vi "EncodersTickCount.vi"() -> (0 "Right ccw  total pulse count":i32, 1 "Left ccw  total pulse count":i32, 2 "Right Motor Pulses per 16 mSec":i32, 3 "Left Motor Pulses per 16 mSec":i32)   [LabVIEW 2013]
doc: "This VI implements the low level control of the motors and sensor for the Starter Kit 2.0 robot. The functionality of this VI is similar to the fixed FPGA personality used by the Starter Kit API."
uses:
  <vilib>/Platform/TimedLoop/XDataNode/timing_clust.ctl
  <vilib>/Platform/TimedLoop/XDataNode/nitl_modes.ctl
  <vilib>/Platform/TimedLoop/XDataNode/wakeup.ctl
  <vilib>/robotics/Utilities/Encoder Count Encoding.ctl
  <vilib>/rvi/Emulation/niFpgaSctlEmulationGetInTimedLoop.vi
  <vilib>/rvi/Emulation/niFpgaEmulationReportErrorSimple.vi
  <vilib>/rvi/Emulation/niFpgaGetClockAttributes.vi
  <vilib>/rvi/Emulation/niFpgaCriticalErrorInLSC.vi
  <vilib>/robotics/Utilities/FPGA Utilities/Count Two Phase Digital Encoder.vi
  Support VIs/Starter Kit 2.0 FPGA Globals.vi
  <vilib>/Platform/TimedLoop/XDataNode/XDataNode.xnode
  <vilib>/robotics/Utilities/NI_Robotics Utilities.lvlib
  <vilib>/Platform/TimedLoop/XDataNode/XDNodeRunTimeDep.lvlib
  <vilib>/robotics/Utilities/FPGA Utilities/NI_Robotics_FPGA Utilities.lvlib
panel:
  in  "stop":bool
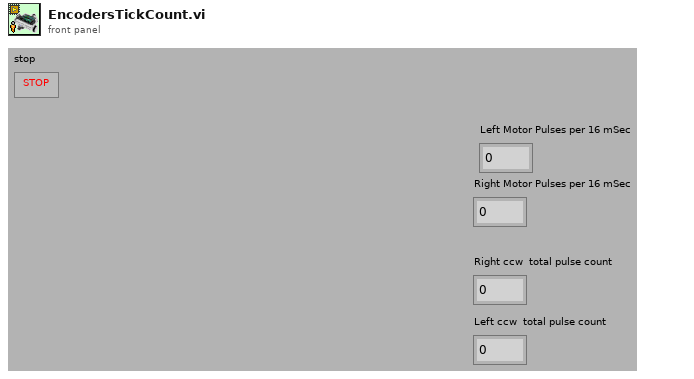
[diagram p1: front panel]
types:
  T1 = typedef "XDNodeRunTimeDep.lvlib/timing_clust.ctl" = cluster{"Expected End [f-1]":u64, "Actual End [f-1]":u64, "Finished Late? [f-1]":bool, "Expected End [i-1]":u64, "Actual End [i-1]":u64, "Finished Late? [i-1]":bool, "Expected Start [i]":u64, "Actual Start [i]":u64, "Expected Start [f]":u64, "Actual Start [f]":u64, "Source Name":string, "Structure Name":string, "Period":i64, "Deadline":i64, "Offset":i64, "Start":i64, "Priority":i32, "Timeout":i32, "Mode":T2, "Wakeup Reason":T3, "Error":errorcluster, "Source Type":string, "Secondary Source Type":string, "Global End Time":u64, "Global Start Time":u64, "Frame Duration":u64, "Iteration Duration":u64, "Assigned CPU":i32, "I/O Scan Engine Mode":u32}
  T2 = typedef "XDNodeRunTimeDep.lvlib/nitl_modes.ctl" = enum32{"No Change", "Process missed periods, maintain original phase", "Discard missed periods, maintain original phase", "Process missed periods, ignore original phase", "Discard missed periods, ignore original phase"}
  T3 = typedef "XDNodeRunTimeDep.lvlib/wakeup.ctl" = enum32{"Normal", "Aborted", "Asynchronous wakeup", "Timing source error", "Timed loop error", "Timeout"}
  T4 = typedef "NI_Robotics Utilities.lvlib/Encoder Count Encoding.ctl" = enum16{"X1", "X2", "X4"}
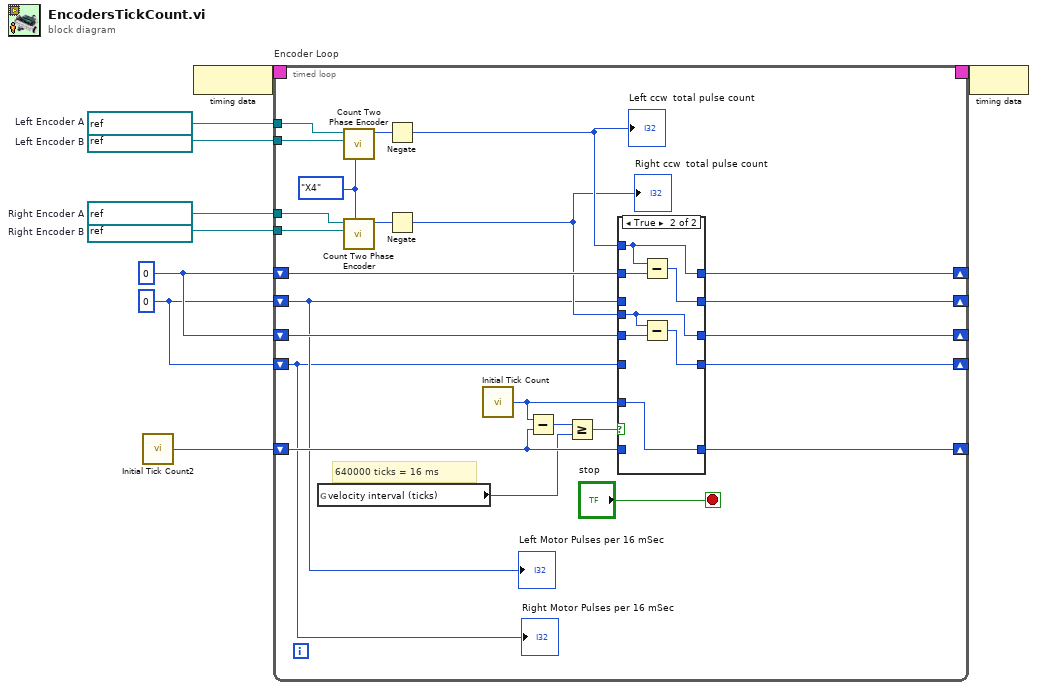
[diagram p0: block diagram]
diagram:
  w1 = refnum<k21> "Port0/DIO3"  # Right Encoder B
  w2 = refnum<k21> "Port0/DIO2"  # Right Encoder A
  w3 = refnum<k21> "Port0/DIO1"  # Left Encoder B
  w4 = refnum<k21> "Port0/DIO0"  # Left Encoder A
  w5 = 0
  w6 = 0 ("Reset Position Value")
  n1 = call "Initial Tick Count2"() -> ("Tick Count(Ticks)"=w7:u32)
  n2 = node-c288() -> (w9:T1)
  n3 = timed-loop "Encoder Loop" {
    timing: w9 -> [_]
    timing-out: [_] -> w8
    shift-right: [w26] -> _
    shift-left: w7 -> [w31]
    shift-right: [w27] -> _
    shift-left: w6 -> [w29]
    shift-right: [w28] -> _
    shift-left: w5 -> [w13]
    shift-right: [w24] -> _
    shift-left: w6 -> [w25]
    shift-right: [w23] -> _
    shift-left: w5 -> [w12]
    tunnel: w4 -> [w20]
    tunnel: w3 -> [w19]
    tunnel: w2 -> [w17]
    tunnel: w1 -> [w16]
    stop <- "stop" stop-if-true
    w14 = Encoder_Count_Encoding."X4" ("count multiplier (X1)")
    # "640000 ticks = 16 ms"
    n4 = global read "Starter Kit 2.0 FPGA Globals.vi" "velocity interval (ticks)"() -> (w11:u32)
    n5 = call-poly <vilib>:"Count Two Phase Encoder.vi"("count encoding (X1)"=w14, "phase B FPGA digital input"=w19, "phase A FPGA digital input"=w20) -> ("new count"=w18:i32)  [unwired: 7 in, 1 out]
    n6 = call-poly <vilib>:"Count Two Phase Encoder.vi"("count encoding (X1)"=w14, "phase B FPGA digital input"=w16, "phase A FPGA digital input"=w17) -> ("new count"=w15:i32)  [unwired: 7 in, 1 out]
    n7 = Negate(x=w18) -> (-x=w22:i32)
    "Left ccw  total pulse count" <- w22
    n8 = Negate(x=w15) -> (-x=w21:i32)
    "Right ccw  total pulse count" <- w21
    n9 = call "Initial Tick Count"() -> ("Tick Count(Ticks)"=w30:u32)
    n10 = Subtract(x=w30, y=w31) -> (x-y=w33:u32)
    n11 = Greater Or Equal?(x=w33, y=w11) -> (x >= y?=w32:bool)
    n12 = case shown="True" w32 {
      tunnel: w30 -> [_ w44]
      tunnel: w31 -> [w38 _]
      tunnel: [w38 w44] -> w26
      tunnel: w29 -> [w37 w45]
      tunnel: [w37 w43] -> w27
      tunnel: w22 -> [_ w43]
      tunnel: [w36 w42] -> w28
      tunnel: w13 -> [w36 _]
      tunnel: w25 -> [w35 w41]
      tunnel: w12 -> [w34 _]
      tunnel: [w35 w40] -> w24
      tunnel: [w34 w39] -> w23
      tunnel: w21 -> [_ w40]
      frame False {
      }
      frame True {
        n13 = Subtract(x=w43, y=w45) -> (x-y=w42:i32)
        n14 = Subtract(x=w40, y=w41) -> (x-y=w39:i32)
      }
    }
    "Left Motor Pulses per 16 mSec" <- w13
    "Right Motor Pulses per 16 mSec" <- w12
  }
  n15 = node-c288(w8) -> ()
